vi "Update Fan State on Sheath Position.vi"(8 "error in":errorcluster, 9 "Init Fan Pos":bool[](array[boolean])=[TRUE, TRUE, TRUE], 10 "Init?":bool, 11 "Servo Switch in":refnum<class "Servo Switch.lvclass">) -> (0 "error out":errorcluster, 3 "Servo Switch out":refnum<class "Servo Switch.lvclass">)   [LabVIEW 2015]
uses:
  Switch/Servo Switch.lvclass
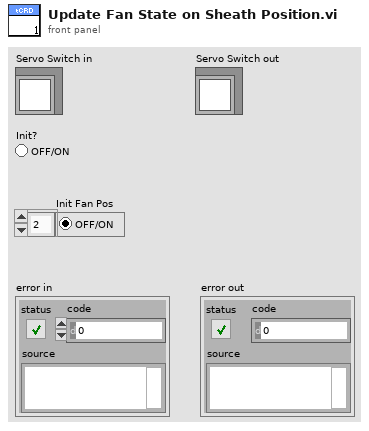
[diagram p1: front panel]
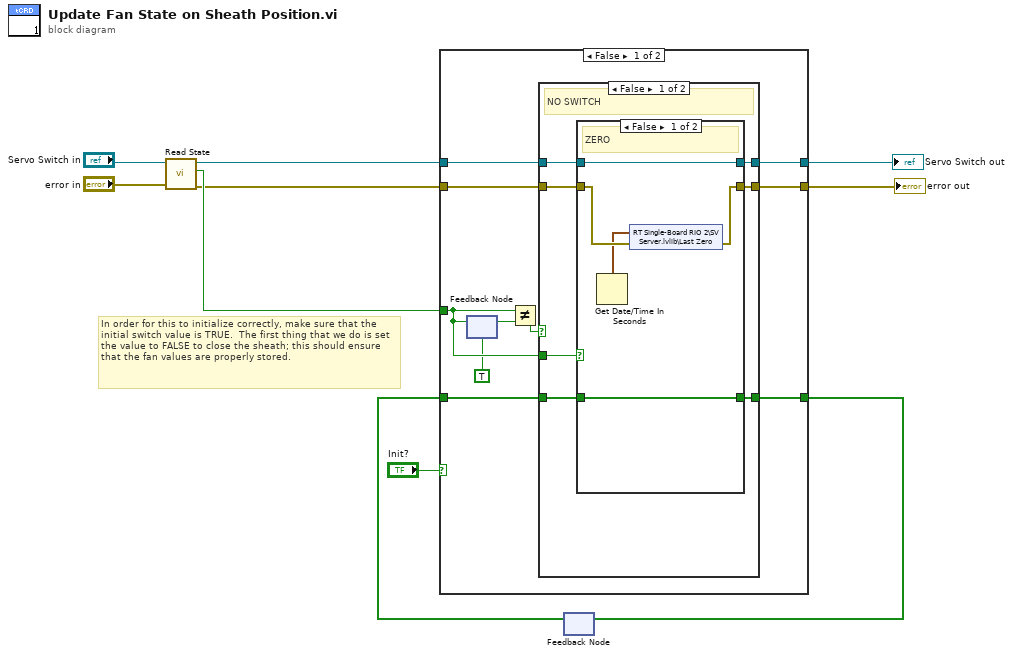
[diagram p0: block diagram]
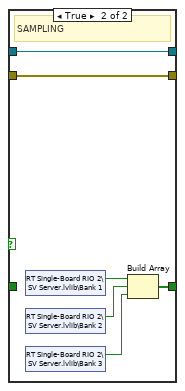
[diagram p2: hidden frame]
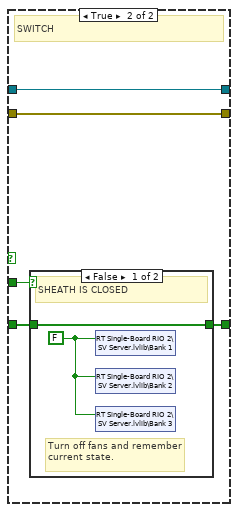
[diagram p3: hidden frame]
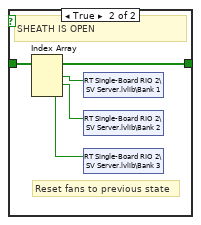
[diagram p4: hidden frame]
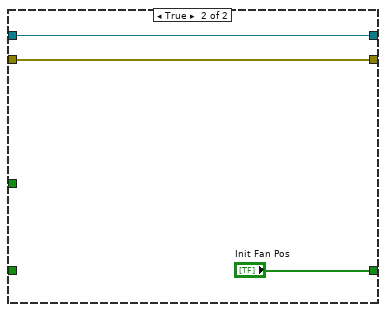
[diagram p5: hidden frame]
diagram:
  # "In order for this to initialize correctly, make sure that the initial switch value is TRUE.  The first thing that we do is set the value to FALSE to close the sheath; this should ensure that the fan values are properly stored."
  n1 = call-dynamic "Read State.vi"("error in (no error)"="error in", "Switch in"="Servo Switch in") -> ("error out"=w3:errorcluster, "State"=w5:bool, "Switch out"=w4:refnum<class "Servo Switch.lvclass">)  [unwired: 7 in]
  n2 = feedback #1() -> (w10:bool[])  [unwired: 1 in]
  n3 = case shown="False" "Init?" {
    tunnel: w10 -> [w20 _]
    tunnel: [w19 "Init Fan Pos"] -> w9
    tunnel: w5 -> [w16 _]
    tunnel: w4 -> [w14 w51]
    tunnel: w3 -> [w13 w50]
    tunnel: [w12 w51] -> w2
    tunnel: [w11 w50] -> w1
    frame False {
      n4 = feedback #2(TRUE ("State")) -> (w18:bool)
      n5 = feedback-in #2(w16) -> ()
      n6 = Not Equal?(x=w16, y=w18) -> (x != y?=w17:bool)
      n7 = case shown="False" w17 {
        tunnel: [w27 w43] -> w19
        tunnel: w20 -> [w25 w42]
        tunnel: w16 -> [w26 w41]
        tunnel: w14 -> [w24 w40]
        tunnel: w13 -> [w23 w39]
        tunnel: [w22 w40] -> w12
        tunnel: [w21 w39] -> w11
        frame False {
          # "NO SWITCH"
          n8 = case shown="False" w26 {
            tunnel: w25 -> [w32 _]
            tunnel: [w32 w35] -> w27
            tunnel: w24 -> [w31 w34]
            tunnel: w23 -> [w30 w33]
            tunnel: [w31 w34] -> w22
            tunnel: [w29 w33] -> w21
            frame False {
              # "ZERO"
              n9 = Get Date/Time In Seconds() -> (seconds since 1Jan1904=w28:timestamp)
              n10 = shared-variable "RT Single-Board RIO 2\\SV Server.lvlib\\Last Zero"(w28, error in=w30) -> (error out=w29:errorcluster)
            }
            frame True {
              # "SAMPLING"
              n11 = shared-variable "RT Single-Board RIO 2\\SV Server.lvlib\\Bank 1"() -> (w38:bool)  [unwired: 1 in, 1 out]
              n12 = shared-variable "RT Single-Board RIO 2\\SV Server.lvlib\\Bank 2"() -> (w37:bool)  [unwired: 1 in, 1 out]
              n13 = shared-variable "RT Single-Board RIO 2\\SV Server.lvlib\\Bank 3"() -> (w36:bool)  [unwired: 1 in, 1 out]
              n14 = Build Array(w38, w37, w36) -> (w35:bool[])
            }
          }
        }
        frame True {
          # "SWITCH"
          n15 = case shown="False" w41 {
            tunnel: [w44 w49] -> w43
            tunnel: w42 -> [w44 w49]
            frame False {
              w45 = FALSE ("Bank 1")
              # "Turn off fans and remember current state."
              # "SHEATH IS CLOSED"
              n16 = shared-variable "RT Single-Board RIO 2\\SV Server.lvlib\\Bank 1"(w45) -> ()  [unwired: 1 in, 1 out]
              n17 = shared-variable "RT Single-Board RIO 2\\SV Server.lvlib\\Bank 2"(w45) -> ()  [unwired: 1 in, 1 out]
              n18 = shared-variable "RT Single-Board RIO 2\\SV Server.lvlib\\Bank 3"(w45) -> ()  [unwired: 1 in, 1 out]
            }
            frame True {
              # "Reset fans to previous state"
              # "SHEATH IS OPEN"
              n19 = Index Array(array=w49) -> (element #1=w48:bool, element #2=w47:bool, element #3=w46:bool)  [unwired: 3 in]
              n20 = shared-variable "RT Single-Board RIO 2\\SV Server.lvlib\\Bank 1"(w48) -> ()  [unwired: 1 in, 1 out]
              n21 = shared-variable "RT Single-Board RIO 2\\SV Server.lvlib\\Bank 2"(w47) -> ()  [unwired: 1 in, 1 out]
              n22 = shared-variable "RT Single-Board RIO 2\\SV Server.lvlib\\Bank 3"(w46) -> ()  [unwired: 1 in, 1 out]
            }
          }
        }
      }
    }
    frame True {
    }
  }
  "error out" <- w1
  "Servo Switch out" <- w2
  n23 = feedback-in #1(w9) -> ()
